vi "Get All Keys By Enumerator.vi"(8 "error in (no error)":errorcluster caption="错误输入（无错误）", 11 "HashTable 输入":refnum<class "HashTable.lvclass"> caption="DNL_LabVIEW Object in") -> (0 "error out":errorcluster caption="错误输出", 2 "Keys":variant[](array[variant]), 3 "HashTable 输出":refnum<class "HashTable.lvclass"> caption="DNL_LabVIEW Object out")   [LabVIEW 2012, in "HashTable.lvclass"]
uses:
  HashTable.lvclass
  Enumerator/Enumerator.lvclass
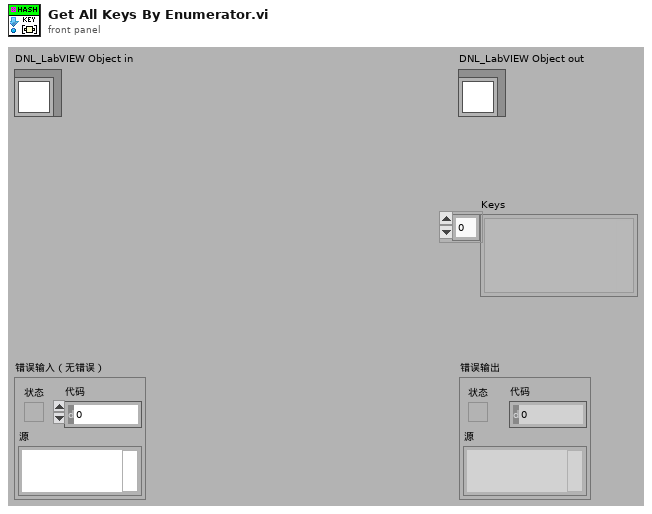
[diagram p1: front panel]
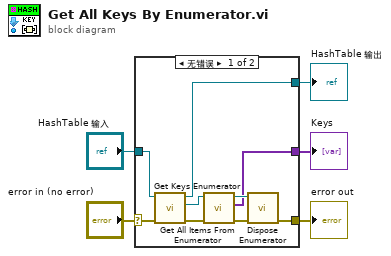
[diagram p0: block diagram]
diagram:
  n1 = case shown="无错误" "error in (no error)" {
    selector: "error in (no error)" -> [w7 w16]
    tunnel: [w6 w16] -> w4
    tunnel: [w8 w15] -> w2
    tunnel: "HashTable 输入" -> [w14 w15]
    tunnel: [w11 _] -> w1
    frame No Error {
      n2 = call "Get Keys Enumerator.vi"("error in (no error)"=w7, "HashTable 输入"=w14) -> ("error out"=w10:errorcluster, "Enumerator 输出"=w13:refnum<class "Enumerator.lvclass">, "HashTable 输出"=w8:refnum<class "HashTable.lvclass">)  [unwired: 7 in]
      n3 = call "Get All Items From Enumerator.vi"("error in (no error)"=w10, "Enumerator 输入"=w13) -> ("error out"=w9:errorcluster, "Items"=w11:variant[], "Enumerator 输出"=w12:refnum<class "Enumerator.lvclass">)  [unwired: 7 in]
      n4 = call "Dispose Enumerator.vi"("error in (no error)"=w9, "Enumerator 输入"=w12) -> ("error out"=w6:errorcluster)  [unwired: 8 in, 1 out]
    }
    frame Error {
    }
  }
  "error out" <- w4
  "HashTable 输出" <- w2
  "Keys" <- w1
